vi "User-Defined Test Advanced.vi"() -> (3 "Unit Test Framework Results":T5)   [LabVIEW 2023]
doc: "Demonstrates how to use the User-defined Test Template.vit file to create an advanced user-defined test VI. This test VI returns not only the test results, but also timing information and details on the output values that do not match given criteria."
uses:
  <vilib>/utf/common/utf_test_result_troll.ctl
  <vilib>/utf/common/utf_test_result.ctl
  <vilib>/utf/common/utf_test_result_failure.ctl
  <vilib>/utf/common/utf_test_comparison_operators.ctl
  <vilib>/utf/common/utf_vi_tag.ctl
  <vilib>/utf/NI_UnitTestFramework.lvlib
panel:
  in  "Unit Test Framework - Result (Parameters)":T1={"result"=enum."Passed", "error message"="", "parameter name"="", "parameter value"=variant, "parameters"=[], "comparison"=enum."=", "requirement ID"="", "VI"=enum."VI under Test", "Used Vector Name"=""}
  # "Overview: Demonstrates how to use the User-defined Test Template.vit file to create an advanced user-defined test VI. This test VI returns not only the test results, but also timing information and details on the output values that do not match given criteria."
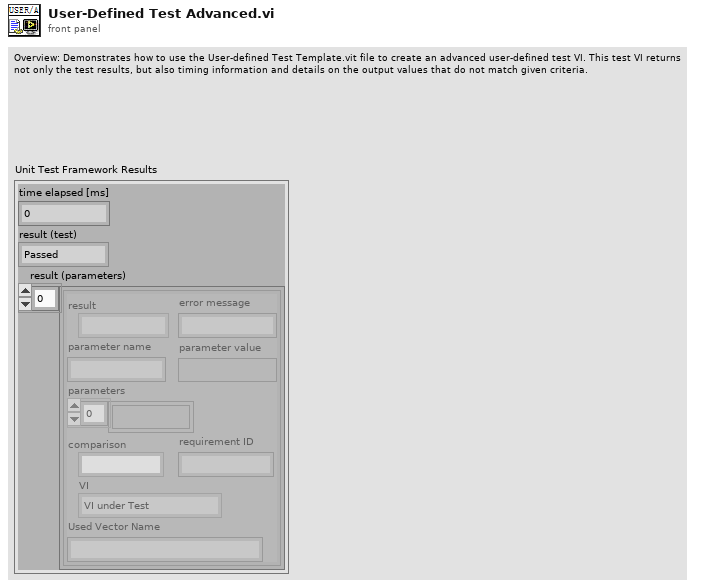
[diagram p1: front panel]
types:
  T1 = typedef "NI_UnitTestFramework.lvlib/utf_test_result_failure.ctl" = cluster{"result":T2, "error message":string, "parameter name":string, "parameter value":variant, "parameters":variant[], "comparison":T3, "requirement ID":string, "VI":T4, "Used Vector Name":string}
  T2 = typedef "NI_UnitTestFramework.lvlib/utf_test_result.ctl" = enum16{"Passed", "Failed", "Error", "Skipped", "Not Processed"}
  T3 = typedef "NI_UnitTestFramework.lvlib/utf_test_comparison_operators.ctl" = enum16{"=", "!=", ">", ">=", "<", "<=", "range", "symmetric tolerance", "asymmetric tolerance", "string contains", "string not contain", "array size", "string length", "array range", "by element", "array range (limit array)", "user-defined", "array contains", "array not contain", "vector length", "= (elm)", "!= (elm)", "= (case insensitive)", "!= (case insensitive)"}
  T4 = typedef "NI_UnitTestFramework.lvlib/utf_vi_tag.ctl" = enum16{"Setup VI", "VI under Test", "Teardown VI"}
  T5 = typedef "NI_UnitTestFramework.lvlib/utf_test_result_troll.ctl" = cluster{"time elapsed [ms]":u32, "result (test)":T2, "result (parameters)":T1[]}
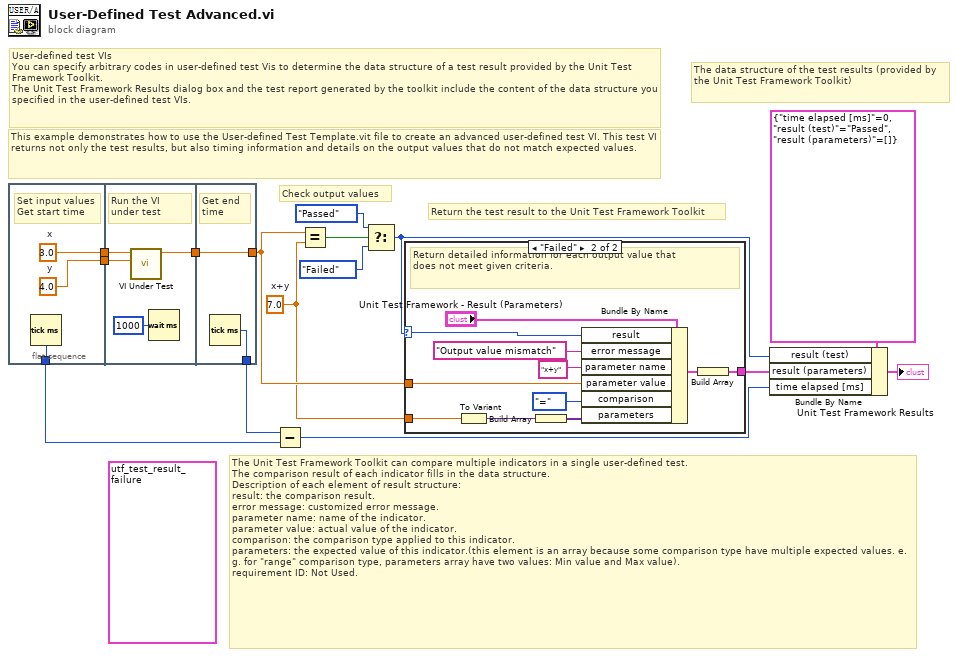
[diagram p0: block diagram]
diagram:
  (unwired) T1 {"result"=enum."Not Processed", "error message"="", "parameter name"="", "parameter value"=variant, "parameters"=[], "comparison"=enum."=", "requirement ID"="", "VI"=enum."VI under Test", "Used Vector Name"=""} ("Unit Test Framework - result (parameters)")
  w1 = 7.0  # x+y
  # "The Unit Test Framework Toolkit can compare multiple indicators in a single user-defined test.\nThe comparison result of each indicator fills in the data structure.\nDescription of each element of result structure:\nresult: the comparison result.\nerror message: customized error message.\nparameter name: name of the indicator.\nparameter value: actual value of the indicator.\ncomparison: the comparison type applied to this indicator.\nparameters: the expected value of this indicator.(this element is an array because some comparison type have multiple expected values. e.g. for \"range\" comparison type, parameters array have two values: Min value and Max value).\nrequirement ID: Not Used."
  # "The data structure of the test results (provided by the Unit Test Framework Toolkit)"
  # "Check output values"
  # "Return the test result to the Unit Test Framework Toolkit"
  # "This example demonstrates how to use the User-defined Test Template.vit file to create an advanced user-defined test VI. This test VI returns not only the test results, but also timing information and details on the output values that do not match expected values."
  # "User-defined test VIs\nYou can specify arbitrary codes in user-defined test Vis to determine the data structure of a test result provided by the Unit Test Framework Toolkit.\nThe Unit Test Framework Results dialog box and the test report generated by the toolkit include the content of the data structure you specified in the user-defined test VIs."
  n1 = flat-sequence {
    tunnel: [w17] -> w10
    tunnel: [w18] -> w9
    tunnel: [w16] -> w4
    tunnel: w10 -> [w20]
    tunnel: w9 -> [w21]
    tunnel: [w22] -> w8
    tunnel: [w24] -> w2
    tunnel: w8 -> [w24]
    tunnel: [w23] -> w5
    frame #0 {
      w17 = 4.0  # y
      w18 = 3.0  # x
      # "Set input values\nGet start time"
      n2 = Tick Count (ms)() -> (millisecond timer value=w16:u32)
    }
    frame #1 {
      # "Run the VI under test"
      n3 = call "VI Under Test.vi"("N2"=w20, "N1"=w21) -> ("Result"=w22:dbl)  [unwired: 1 in, 8 out]
      n4 = Wait (ms)(milliseconds to wait=u32 1000) -> ()  [unwired: 1 out]
    }
    frame #2 {
      # "Get end time"
      n5 = Tick Count (ms)() -> (millisecond timer value=w23:u32)
    }
  }
  n6 = Subtract(x=w5, y=w4) -> (x-y=w3:u32)
  n7 = Equal?(x=w2, y=w1) -> (x = y?=w14:bool)
  n8 = Select(t=utf_test_result."Passed" ("Result (Test)"), s=w14, f=utf_test_result."Failed" ("Result (Test)")) -> (s? t:f=w7:T2)
  n9 = case shown="\"Failed\"" w7 {
    selector: w7 -> [_ w34]
    tunnel: w2 -> [_ w31]
    tunnel: [_ w28] -> w6
    tunnel: w1 -> [_ w27]
    frame "Passed", Default {
      # "Do not return any detailed information if the test has passed."
    }
    frame "Failed" {
      # "Return detailed information for each output value that\ndoes not meet given criteria."
      n10 = To Variant(anything=w27) -> (Variant=w26:variant)
      n11 = Build Array(w26) -> (w25:variant[])
      n12 = Bundle By Name(cluster="Unit Test Framework - Result (Parameters)", "result"=w34, "error message"="Output value mismatch", "parameter name"="x+y", "parameter value"=w31, "comparison"=utf_test_comparison_operators."=" ("Comparison"), "parameters"=w25) -> (w29:T1)
      n13 = Build Array(w29) -> (w28:T1[])
    }
  }
  n14 = Bundle By Name(cluster=T5 {"time elapsed [ms]"=0, "result (test)"=enum."Passed", "result (parameters)"=[]} ("Unit Test Framework - Result"), "result (test)"=w7, "result (parameters)"=w6, "time elapsed [ms]"=w3) -> (→"Unit Test Framework Results":T5)
